vi "Shooter Loop.vi"(1 "MotorControlDevRef":T1={"DeviceStatus"={"status"=FALSE, "code"=0, "source"=""}, "Type"=enum."PWM", "PWM"={"Digital Module"=enum."Digital Module 1", "PWM Channel"=enum."Invalid", "DeadBand"={"Name"="", "maxPositivePwm"=0, "minPositivePwm"=0, "centerPwm"=0, "maxNegativePwm"=0, "minNegativePwm"=0, "angularRange"=0}}, "CAN"={"Device Number"=0, "Control Mode"=enum."Percent VBus", "Semaphore"=refnum, "Max Vout"=12.0}, "Invert"=FALSE, "TransformRef"=refnum, "InvTransformRef"=refnum}, 2 "CounterDevRef":T8={"DevStatus"={"status"=FALSE, "code"=0, "source"=""}, "CntIndex"=enum."Invalid"}) -> ()   [LabVIEW 2012]
uses:
  <vilib>/Rock Robotics/WPI/Counter/WPI_CounterDevRef.ctl
  <vilib>/Rock Robotics/SystemInterfaces/Counter/FPGA_CounterCtrSystemIndex.ctl
  <vilib>/Rock Robotics/WPI/MotorControl/WPI_MotorControlDeviceRef.ctl
  <vilib>/Rock Robotics/SystemInterfaces/Typedef/FPGA_TypedefDigitalModule.ctl
  <vilib>/Rock Robotics/SystemInterfaces/DIO/FPGA_DIOPWMChannel.ctl
  <vilib>/Rock Robotics/WPI/PWM/WPI_PWMDeadband.ctl
  <vilib>/Rock Robotics/WPI/CAN/Jaguar/SubVIs/WPI_CANJaguar_ControlMode.ctl
  <vilib>/Rock Robotics/WPI/PWM/WPI_PWMTransform_ConPane.ctl
panel:
  in  "Stab Auto":bool=TRUE
  out "RPM Stable ?":bool
  in  "Shooter Stable Tol (sec)":dbl(knob)=0.4038944862363681 scale=0.0..1.0
  in  "Test?":bool
  in  "Shooter Motor RPM":dbl(knob)=0.006611706614844206 scale=0.0..5000.0
  out "Motor Control":cluster{"ShooterRpmControl":dbl, "RPM":dbl}(graph)
  out "Motor Command":dbl(slide) scale=0.0..1.0
  out "RPM":dbl
  in  "TBH ?":bool=TRUE
  out "Period (sec)":dbl
  in  "TBH Gain":dbl(knob)=3.037792394667692e-05 scale=0.0..0.0001
  out "RPM In Tol?":bool
  in  "Tol":dbl(knob)=175.82084414799198 scale=0.0..400.0
  in  "s":bool
  out "RPM In Tol ?":bool
  # "Take Back Half"
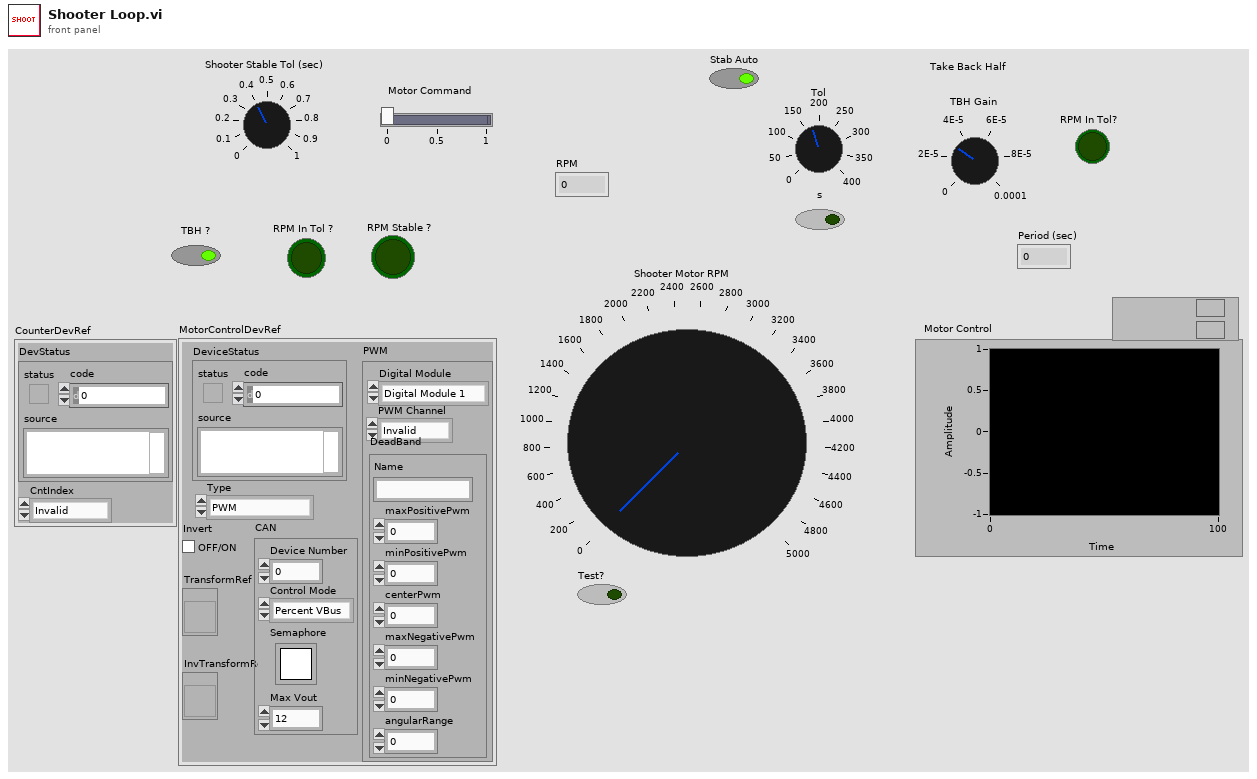
[diagram p1: front panel]
types:
  T1 = typedef "WPI_MotorControlDeviceRef.ctl" = cluster{"DeviceStatus":errorcluster, "Type":enum16{"PWM", "CAN"}, "PWM":cluster{"Digital Module":T2, "PWM Channel":T3, "DeadBand":T4}, "CAN":cluster{"Device Number":u8, "Control Mode":T5, "Semaphore":T6, "Max Vout":dbl}, "Invert":bool, "TransformRef":T7, "InvTransformRef":T7}
  T2 = typedef "FPGA_TypedefDigitalModule.ctl" = enum16{"Digital Module 1", "Digital Module 2"}
  T3 = typedef "FPGA_DIOPWMChannel.ctl" = enum8{"PWM 1", "PWM 2", "PWM 3", "PWM 4", "PWM 5", "PWM 6", "PWM 7", "PWM 8", "PWM 9", "PWM 10", "Invalid"}
  T4 = typedef "WPI_PWMDeadband.ctl" = cluster{"Name":string, "maxPositivePwm":i32, "minPositivePwm":i32, "centerPwm":i32, "maxNegativePwm":i32, "minNegativePwm":i32, "angularRange":u16}
  T5 = typedef "WPI_CANJaguar_ControlMode.ctl" = enum8{"Percent VBus", "Current", "Speed", "Position", "Voltage"}
  T6 = typedef "Semaphore RefNum" = refnum<k1>
  T7 = typedef "WPI_PWMTransform_ConPane.ctl" = refnum<vi>
  T8 = typedef "WPI_CounterDevRef.ctl" = cluster{"DevStatus":errorcluster, "CntIndex":T9}
  T9 = typedef "FPGA_CounterCtrSystemIndex.ctl" = enum8{"Ctr 0", "Ctr 1", "Ctr 2", "Ctr 3", "Ctr 4", "Ctr 5", "Ctr 6", "Ctr 7", "Invalid"}
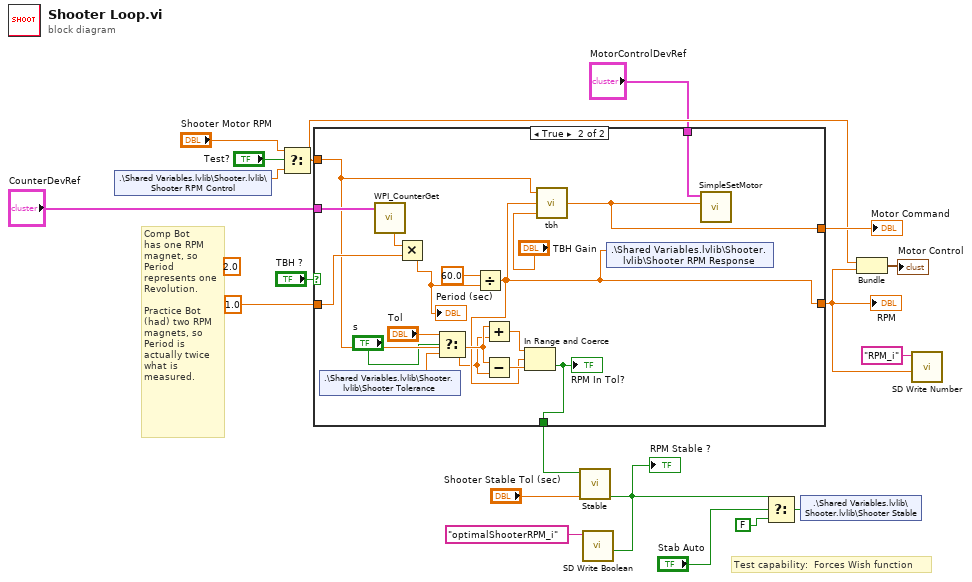
[diagram p0: block diagram]
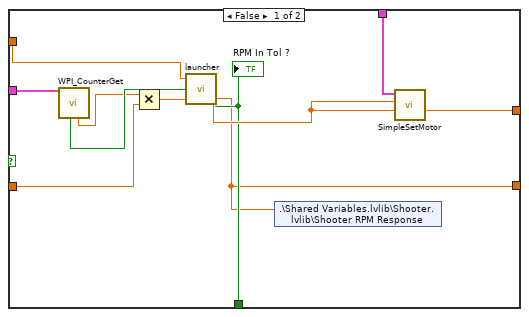
[diagram p2: hidden frame]
diagram:
  (unwired) 2.0 ("t")
  # "Test capability:  Forces Wish function"
  # "Comp Bot\nhas one RPM \nmagnet, so\nPeriod\nrepresents one\nRevolution.\n\nPractice Bot\n(had) two RPM\nmagnets, so\nPeriod is\nactually twice\nwhat is\nmeasured."
  n1 = shared-variable ".\\Shared Variables.lvlib\\Shooter.lvlib\\Shooter RPM Control"() -> (w5:dbl)  [unwired: 1 in, 1 out]
  n2 = Select(t="Shooter Motor RPM", s="Test?", f=w5) -> (s? t:f=w13:dbl)
  n3 = case shown="True" "TBH ?" {
    tunnel: "MotorControlDevRef" -> [w29 w44]
    tunnel: "CounterDevRef" -> [w27 w46]
    tunnel: [w26 w39] -> w18
    tunnel: [w20 w32] -> w16
    tunnel: 1.0 ("t") -> [w23 w42]
    tunnel: w13 -> [w22 w35]
    tunnel: [w21 w36] -> w10
    frame False {
      n4 = call <vilib>:"WPI_CounterGet.vi"("CounterDevRef in"=w27) -> ("Period (sec)"=w24:dbl, "Stopped"=w28:bool)  [unwired: 5 in, 4 out]
      n5 = Multiply(x=w24, y=w23) -> (x*y=w25:dbl)
      n6 = call "launcher.vi"("RPM Control"=w22, "Stall"=w28, "Period (sec)"=w25) -> ("RPM"=w20:dbl, "RPM In Tol?"=w21:bool, "Motor Output"=w26:dbl)  [unwired: 2 in]
      "RPM In Tol ?" <- w21
      n7 = shared-variable ".\\Shared Variables.lvlib\\Shooter.lvlib\\Shooter RPM Response"(w20) -> ()  [unwired: 1 in, 1 out]
      n8 = call "SimpleSetMotor.vi"("Output"=w26, "MotorControlDevRef"=w29) -> ()  [unwired: 8 in, 2 out]
    }
    frame True {
      n9 = shared-variable ".\\Shared Variables.lvlib\\Shooter.lvlib\\Shooter Tolerance"() -> (w31:dbl)  [unwired: 1 in, 1 out]
      n10 = call <vilib>:"WPI_CounterGet.vi"("CounterDevRef in"=w46) -> ("Period (sec)"=w43:dbl)  [unwired: 5 in, 5 out]
      n11 = Multiply(x=w43, y=w42) -> (x*y=w41:dbl)
      "Period (sec)" <- w41
      n12 = Select(t="Tol", s="s", f=w31) -> (s? t:f=w30:dbl)
      n13 = Divide(x=60.0, y=w41) -> (x/y=w32:dbl)
      n14 = Add(x=w35, y=w30) -> (x+y=w38:dbl)
      n15 = Subtract(x=w35, y=w30) -> (x-y=w37:dbl)
      n16 = In Range and Coerce(upper limit=w38, x=w32, lower limit=w37) -> (In Range?=w36:bool)  [unwired: 1 out]
      "RPM In Tol?" <- w36
      n17 = call "tbh.vi"("Gain"="TBH Gain", "Act"=w32, "Cmd"=w35) -> ("Out"=w39:dbl)
      n18 = shared-variable ".\\Shared Variables.lvlib\\Shooter.lvlib\\Shooter RPM Response"(w32) -> ()  [unwired: 1 in, 1 out]
      n19 = call "SimpleSetMotor.vi"("Output"=w39, "MotorControlDevRef"=w44) -> ()  [unwired: 8 in, 2 out]
    }
  }
  "RPM" <- w16
  "Motor Command" <- w18
  n20 = call "Stable.vi"("Eval Period (sec)"="Shooter Stable Tol (sec)", "Signal Input"=w10) -> ("Stable"=w7:bool)  [unwired: 9 in]
  "RPM Stable ?" <- w7
  n21 = call <vilib>:"SD Write Boolean.vi"("Boolean"=w7, "Name"="optimalShooterRPM_i") -> ()  [unwired: 8 in, 2 out]
  n22 = Select(t=w7, s="Stab Auto", f=FALSE) -> (s? t:f=w4:bool)
  n23 = shared-variable ".\\Shared Variables.lvlib\\Shooter.lvlib\\Shooter Stable"(w4) -> ()  [unwired: 1 in, 1 out]
  n24 = Bundle("Double"=w13, "RPM"=w16) -> (→"Motor Control":cluster{"Double":dbl, "RPM":dbl})  [unwired: 1 in]
  n25 = call <vilib>:"SD Write Number.vi"("Numeric"=w16, "Name"="RPM_i") -> ()  [unwired: 8 in, 2 out]
